vi "Watermark Position.vi"(0 "Watermark Cluster IN":T3={"Show? (F)"=TRUE, "Type"=enum."Image", "Opacity (%)"=10.0, "Rotate(°)"=0.0, "Position"={"Position"=enum."Center (text section)", "X"=0.0, "Y"=0.0}, "Image path"=path "", "Scaled(%)"=100.0, "Image refnum"=refnum, "Text"="CONFIDENTIAL", "Font"={"Name"="", "Size"=-1.0, "Color"=0}, "Font refnum"=refnum, "Alignment"=enum."Center", "Automatic"=FALSE}, 7 "Page dimensions":T1={"Start at page"=1, "Orientation"=enum."Portrait", "widht"=612.0, "height"=792.0, "Margin left"=72.0, "Margin right"=72.0, "Margin top"=72.0, "Margin bottom"=72.0}, 11 "error in (no error)":errorcluster) -> (4 "Watermark Cluster OUT":T3={"Show? (F)"=TRUE, "Type"=enum."Image", "Opacity (%)"=10.0, "Rotate(°)"=0.0, "Position"={"Position"=enum."Center (text section)", "X"=0.0, "Y"=0.0}, "Image path"=path "", "Scaled(%)"=100.0, "Image refnum"=refnum, "Text"="CONFIDENTIAL", "Font"={"Name"="", "Size"=-1.0, "Color"=0}, "Font refnum"=refnum, "Alignment"=enum."Center", "Automatic"=FALSE}, 6 "Box":cluster{"width":sgl, "height":sgl}, 8 "Hypothenus":sgl, 10 "Angle (rad)":dbl, 15 "error out":errorcluster)   [LabVIEW 2012]
doc: "Version 1.0\nDeveloped by Jean-Marc Simard\nCopyright © 2010, Exaprom Inc.\nAll rights reserved.\nLicense: BSD\n\nWith iTextSharp 4.1.6 (http://itextsharp.sourceforge.net)\nunder Mozilla Public License Version 1.1\n(http://www.mozilla.org/MPL/MPL-1.1.html)"
uses:
  Controls/Watermark cluster2.ctl
  Controls/Watermark Position.ctl
  C:/Users/MaxCorp/Documents/TopPerm - Base/DLL/itextsharp.dll
  DLL/itextsharp.dll
  Controls/Font size.ctl
  Controls/Font color.ctl
  Controls/Header footer horiz alignment.ctl
  Controls/Page dimensions.ctl
  Controls/Page Orientation.ctl
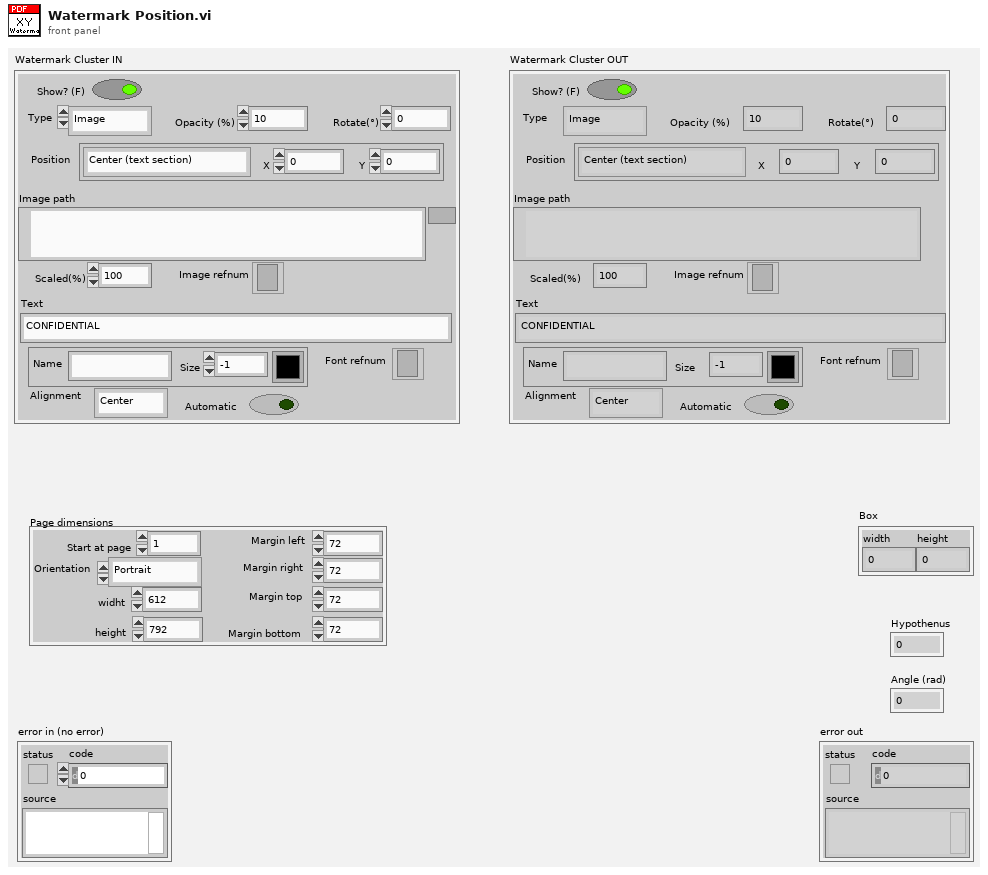
[diagram p1: front panel]
types:
  T1 = typedef "Page dimensions.ctl" = cluster{"Start at page":i32, "Orientation":T2, "widht":sgl, "height":sgl, "Margin left":sgl, "Margin right":sgl, "Margin top":sgl, "Margin bottom":sgl}
  T2 = typedef "Page Orientation.ctl" = enum16{"Portrait", "Landscape"}
  T3 = typedef "Watermark cluster2.ctl" = cluster{"Show? (F)":bool, "Type":enum16{"Image", "Text"}, "Opacity (%)":sgl, "Rotate(°)":sgl, "Position":cluster{"Position":T4, "X":sgl, "Y":sgl}, "Image path":path, "Scaled(%)":sgl, "Image refnum":refnum<k24>, "Text":string, "Font":cluster{"Name":string, "Size":T5, "Color":T6}, "Font refnum":refnum<k24>, "Alignment":T7, "Automatic":bool}
  T4 = typedef "Watermark Position.ctl" = enum16{"Absolute", "Center (page)", "Center (text section)"}
  T5 = typedef "Font size.ctl" = sgl
  T6 = typedef "Font color.ctl" = u32
  T7 = typedef "Header footer horiz alignment.ctl" = enum16{"Left", "Center", "Right"}
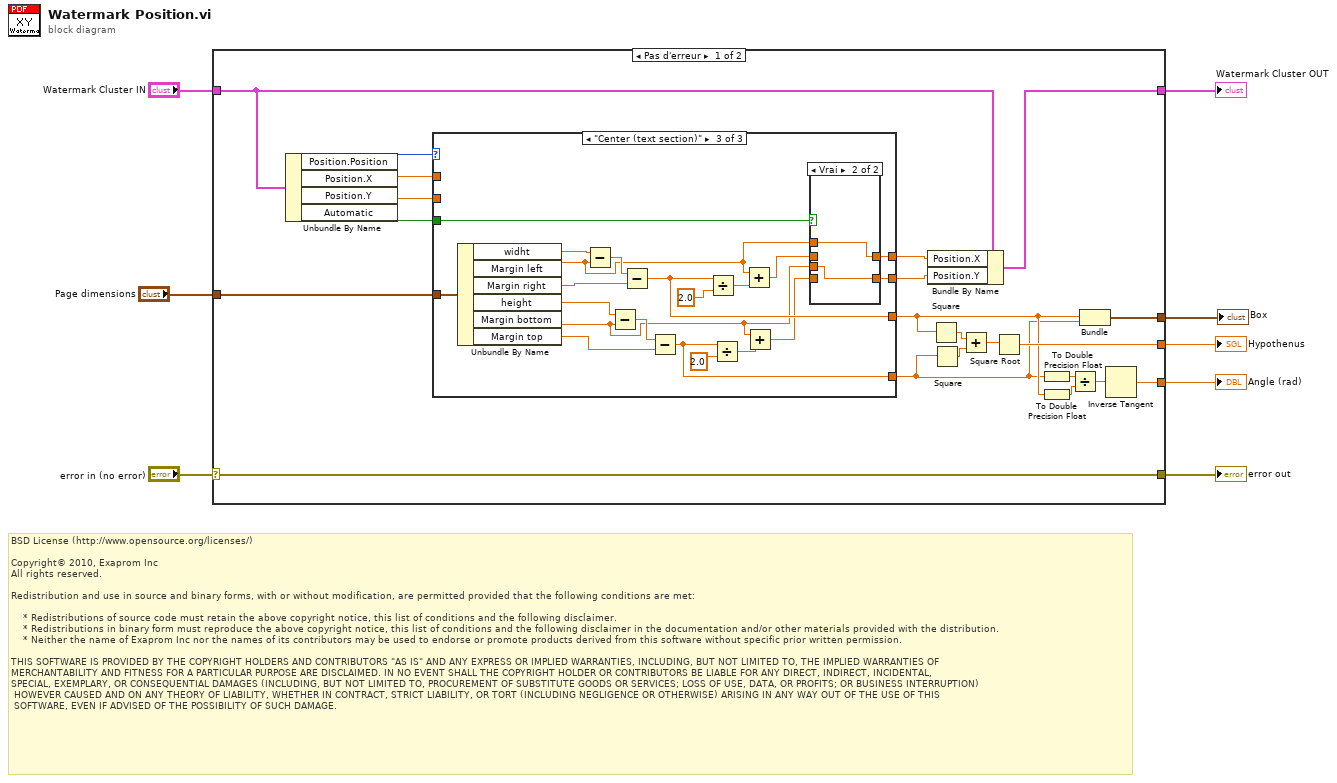
[diagram p0: block diagram]
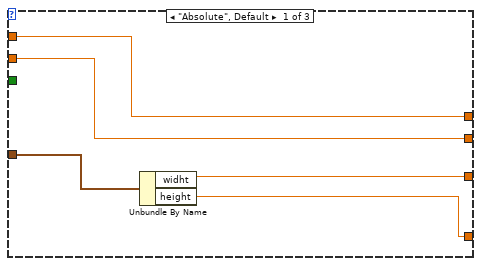
[diagram p2: hidden frame]
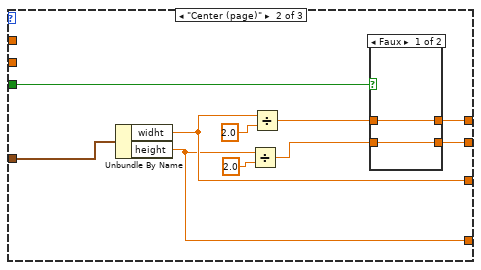
[diagram p3: hidden frame]
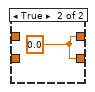
[diagram p4: hidden frame]
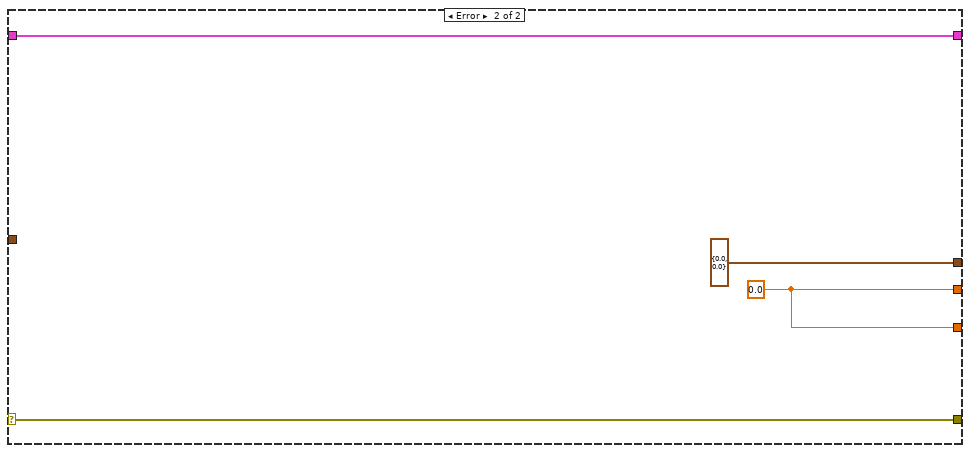
[diagram p6: hidden frame]
diagram:
  # "BSD License (http://www.opensource.org/licenses/)\n\nCopyright© 2010, Exaprom Inc\nAll rights reserved.\n\nRedistribution and use in source and binary forms, with or without modification, are permitted provided that the following conditions are met:\n\n    * Redistributions of source code must retain the above copyright notice, this list of conditions and the following disclaimer.\n    * Redistributions in binary form must reproduce the above copyright notice, this list of conditions and the following disclaimer in the documentation and/or other materials provided with the distribution.\n    * Neither the name of Exaprom Inc nor the names of its contributors may be used to endorse or promote products derived from this software without specific prior written permission.\n\nTHIS SOFTWARE IS PROVIDED BY THE COPYRIGHT HOLDERS AND CONTRIBUTORS \"AS IS\" AND ANY EXPRESS OR IMPLIED WARRANTIES, INCLUDING, BUT NOT LIMITED TO, THE IMPLIED WARRANTIES OF \nMERCHANTABILITY AND FITNESS FOR A PARTICULAR PURPOSE ARE DISCLAIMED. IN NO EVENT SHALL THE COPYRIGHT HOLDER OR CONTRIBUTORS BE LIABLE FOR ANY DIRECT, INDIRECT, INCIDENTAL,\nSPECIAL, EXEMPLARY, OR CONSEQUENTIAL DAMAGES (INCLUDING, BUT NOT LIMITED TO, PROCUREMENT OF SUBSTITUTE GOODS OR SERVICES; LOSS OF USE, DATA, OR PROFITS; OR BUSINESS INTERRUPTION)\n HOWEVER CAUSED AND ON ANY THEORY OF LIABILITY, WHETHER IN CONTRACT, STRICT LIABILITY, OR TORT (INCLUDING NEGLIGENCE OR OTHERWISE) ARISING IN ANY WAY OUT OF THE USE OF THIS\n SOFTWARE, EVEN IF ADVISED OF THE POSSIBILITY OF SUCH DAMAGE."
  n1 = case shown="Pas d'erreur" "error in (no error)" {
    selector: "error in (no error)" -> [w29 w75]
    tunnel: [w29 w75] -> w8
    tunnel: "Page dimensions" -> [w23 _]
    tunnel: [w18 w74] -> w5
    tunnel: "Watermark Cluster IN" -> [w19 w74]
    tunnel: [w16 w73] -> w3
    tunnel: [w15 w73] -> w2
    tunnel: [w12 cluster{"widht":sgl, "height":sgl} {"widht"=0.0, "height"=0.0}] -> w1
    frame No Error {
      n2 = Unbundle By Name(w19) -> ("Position.Position"=w22:T4, "Position.X"=w21:sgl, "Position.Y"=w20:sgl, "Automatic"=w11:bool)
      n3 = case shown="\"Center (text section)\"" w22 {
        tunnel: w23 -> [w32 w44 w57]
        tunnel: [w34 w38 w52] -> w28
        tunnel: w21 -> [w34 _ _]
        tunnel: [w33 w37 w50] -> w27
        tunnel: w20 -> [w33 _ _]
        tunnel: [w31 w41 w56] -> w14
        tunnel: [w30 w40 w55] -> w13
        tunnel: w11 -> [_ w39 w54]
        frame "Absolute", Default {
          n4 = Unbundle By Name(w32) -> ("widht"=w31:sgl, "height"=w30:sgl)
        }
        frame "Center (page)" {
          n5 = Unbundle By Name(w44) -> ("widht"=w41:sgl, "height"=w40:sgl)
          n6 = Divide(x=w40, y=sgl 2.0) -> (x/y=w35:sgl)
          n7 = Divide(x=w41, y=sgl 2.0) -> (x/y=w36:sgl)
          n8 = case shown="Faux" w39 {
            tunnel: [w46 w47] -> w38
            tunnel: [w45 w47] -> w37
            tunnel: w36 -> [w46 _]
            tunnel: w35 -> [w45 _]
            frame False {
            }
            frame True {
              w47 = sgl 0.0 ("X")
            }
          }
        }
        frame "Center (text section)" {
          n9 = Unbundle By Name(w57) -> ("widht"=w60:sgl, "Margin left"=w49:sgl, "Margin right"=w61:sgl, "height"=w66:sgl, "Margin bottom"=w48:sgl, "Margin top"=w67:sgl)
          n10 = Subtract(x=w60, y=w49) -> (x-y=w59:sgl)
          n11 = Subtract(x=w66, y=w48) -> (x-y=w64:sgl)
          n12 = Subtract(x=w59, y=w61) -> (x-y=w56:sgl)
          n13 = Subtract(x=w64, y=w67) -> (x-y=w55:sgl)
          n14 = Divide(x=w56, y=sgl 2.0) -> (x/y=w62:sgl)
          n15 = Divide(x=w55, y=sgl 2.0) -> (x/y=w63:sgl)
          n16 = Add(x=w49, y=w62) -> (x+y=w53:sgl)
          n17 = Add(x=w48, y=w63) -> (x+y=w51:sgl)
          n18 = case shown="Vrai" w54 {
            tunnel: w53 -> [w69 _]
            tunnel: [w69 w71] -> w52
            tunnel: w51 -> [w68 _]
            tunnel: [w68 w70] -> w50
            tunnel: w49 -> [_ w71]
            tunnel: w48 -> [_ w70]
            frame False {
            }
            frame True {
            }
          }
        }
      }
      n19 = Bundle By Name(cluster=w19, "Position.X"=w28, "Position.Y"=w27) -> (w18:T3)
      n20 = Square(x=w14) -> (x^2=w25:sgl)
      n21 = Square(x=w13) -> (x^2=w26:sgl)
      n22 = Add(x=w25, y=w26) -> (x+y=w24:sgl)
      n23 = Square Root(x=w24) -> (sqrt(x)=w16:sgl)
      n24 = To Double Precision Float(number=w13) -> (double precision float=w10:dbl)
      n25 = To Double Precision Float(number=w14) -> (double precision float=w9:dbl)
      n26 = Divide(x=w10, y=w9) -> (x/y=w17:dbl)
      n27 = Bundle("widht"=w14, "height"=w13) -> (w12:cluster{"widht":sgl, "height":sgl})  [unwired: 1 out]
      n28 = Inverse Tangent(1:w17) -> (0:w15:dbl)
    }
    frame Error {
      w73 = sgl 0.0
    }
  }
  "error out" <- w8
  "Watermark Cluster OUT" <- w5
  "Hypothenus" <- w3
  "Angle (rad)" <- w2
  "Box" <- w1
